vi "Demo.vi"() -> ()   [LabVIEW 2018]
uses:
  SquidstatStructures/AisDCData.ctl
  SquidstatStructures/AisACData.ctl
panel:
  in  "Start Experiment":bool
  in  "Experiment To Run":enum32{"DC Experiment", "AC Experiment"}(radio)
  out "Device Initialized?":bool
  in  "Channel To Run":i32
  in  "Stop Experiment":bool
  out "Experiment Active?":bool
  out "Last Channel":dbl
  out "Last AC Data":T1
  out "Last DC Data":T2
  out "Step Number":i32
  out "Step Name":string
  in  "Device Name":string
  # "Controls"
  # "Indicators"
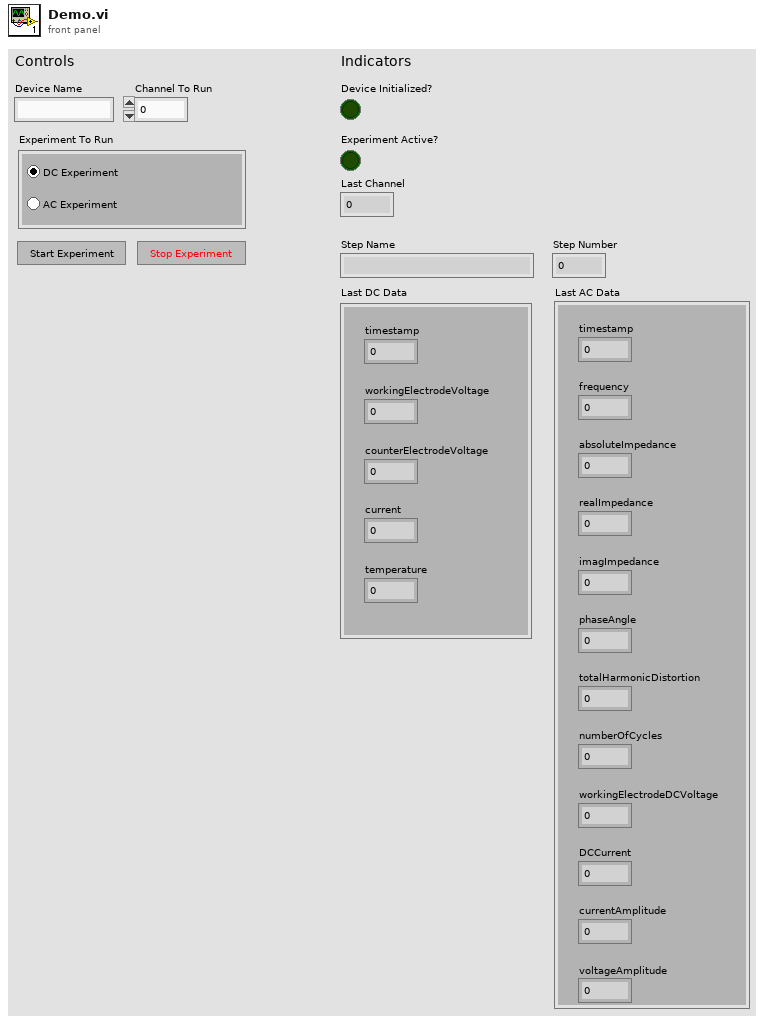
[diagram p1: front panel]
types:
  T1 = typedef "AisACData.ctl" = cluster{"timestamp":dbl, "frequency":dbl, "absoluteImpedance":dbl, "realImpedance":dbl, "imagImpedance":dbl, "phaseAngle":dbl, "totalHarmonicDistortion":dbl, "numberOfCycles":dbl, "workingElectrodeDCVoltage":dbl, "DCCurrent":dbl, "currentAmplitude":dbl, "voltageAmplitude":dbl}
  T2 = typedef "AisDCData.ctl" = cluster{"timestamp":dbl, "workingElectrodeVoltage":dbl, "counterElectrodeVoltage":dbl, "current":dbl, "temperature":dbl}
  T3 = typedef "AisUserEvents.ctl" = cluster{"Disconnected":refnum<user-event>, "Ground State":refnum<user-event>, "Device Error":refnum<user-event>, "New Element Started":refnum<user-event>, "Experiment Stopped":refnum<user-event>, "Experiment Paused":refnum<user-event>, "Experiment Resumed":refnum<user-event>, "DC Data":refnum<user-event>, "AC Data":refnum<user-event>}
  T4 = typedef "AisExperimentNode.ctl" = cluster{"Step Name":cluster{"char":u8, "char 2":u8, "char 3":u8, "char 4":u8, "char 5":u8, "char 6":u8, "char 7":u8, "char 8":u8, "char":u8, "char 9":u8, "char 10":u8, "char 11":u8, "char 12":u8, "char 13":u8, "char 14":u8, "char 15":u8, "char 16":u8, "char 17":u8, "char 18":u8, "char 19":u8, "char 20":u8, "char 21":u8, "char 22":u8, "char 23":u8, "char 24":u8, "char 25":u8, "char 26":u8, "char 27":u8, "char 28":u8, "char 29":u8, "char 30":u8, "char 31":u8, "char 32":u8, "char 33":u8, "char 34":u8, "char 35":u8, "char 36":u8, "char 37":u8, "char 38":u8, "char 39":u8, "char 40":u8, "char 41":u8, "char 42":u8, "char 43":u8, "char 44":u8, "char 45":u8, "char 46":u8, "char 47":u8, "char 48":u8, "char 49":u8, "char 50":u8, "char 50":u8}, "Step Number":i32, "Substep Number":i32, "Cycle Number":i32}
  T5 = cluster{"char":u8, "char 2":u8, "char 3":u8, "char 4":u8, "char 5":u8, "char 6":u8, "char 7":u8, "char 8":u8, "char":u8, "char 9":u8, "char 10":u8, "char 11":u8, "char 12":u8, "char 13":u8, "char 14":u8, "char 15":u8, "char 16":u8, "char 17":u8, "char 18":u8, "char 19":u8, "char 20":u8, "char 21":u8, "char 22":u8, "char 23":u8, "char 24":u8, "char 25":u8, "char 26":u8, "char 27":u8, "char 28":u8, "char 29":u8, "char 30":u8, "char 31":u8, "char 32":u8, "char 33":u8, "char 34":u8, "char 35":u8, "char 36":u8, "char 37":u8, "char 38":u8, "char 39":u8, "char 40":u8, "char 41":u8, "char 42":u8, "char 43":u8, "char 44":u8, "char 45":u8, "char 46":u8, "char 47":u8, "char 48":u8, "char 49":u8, "char 50":u8, "char 50":u8}
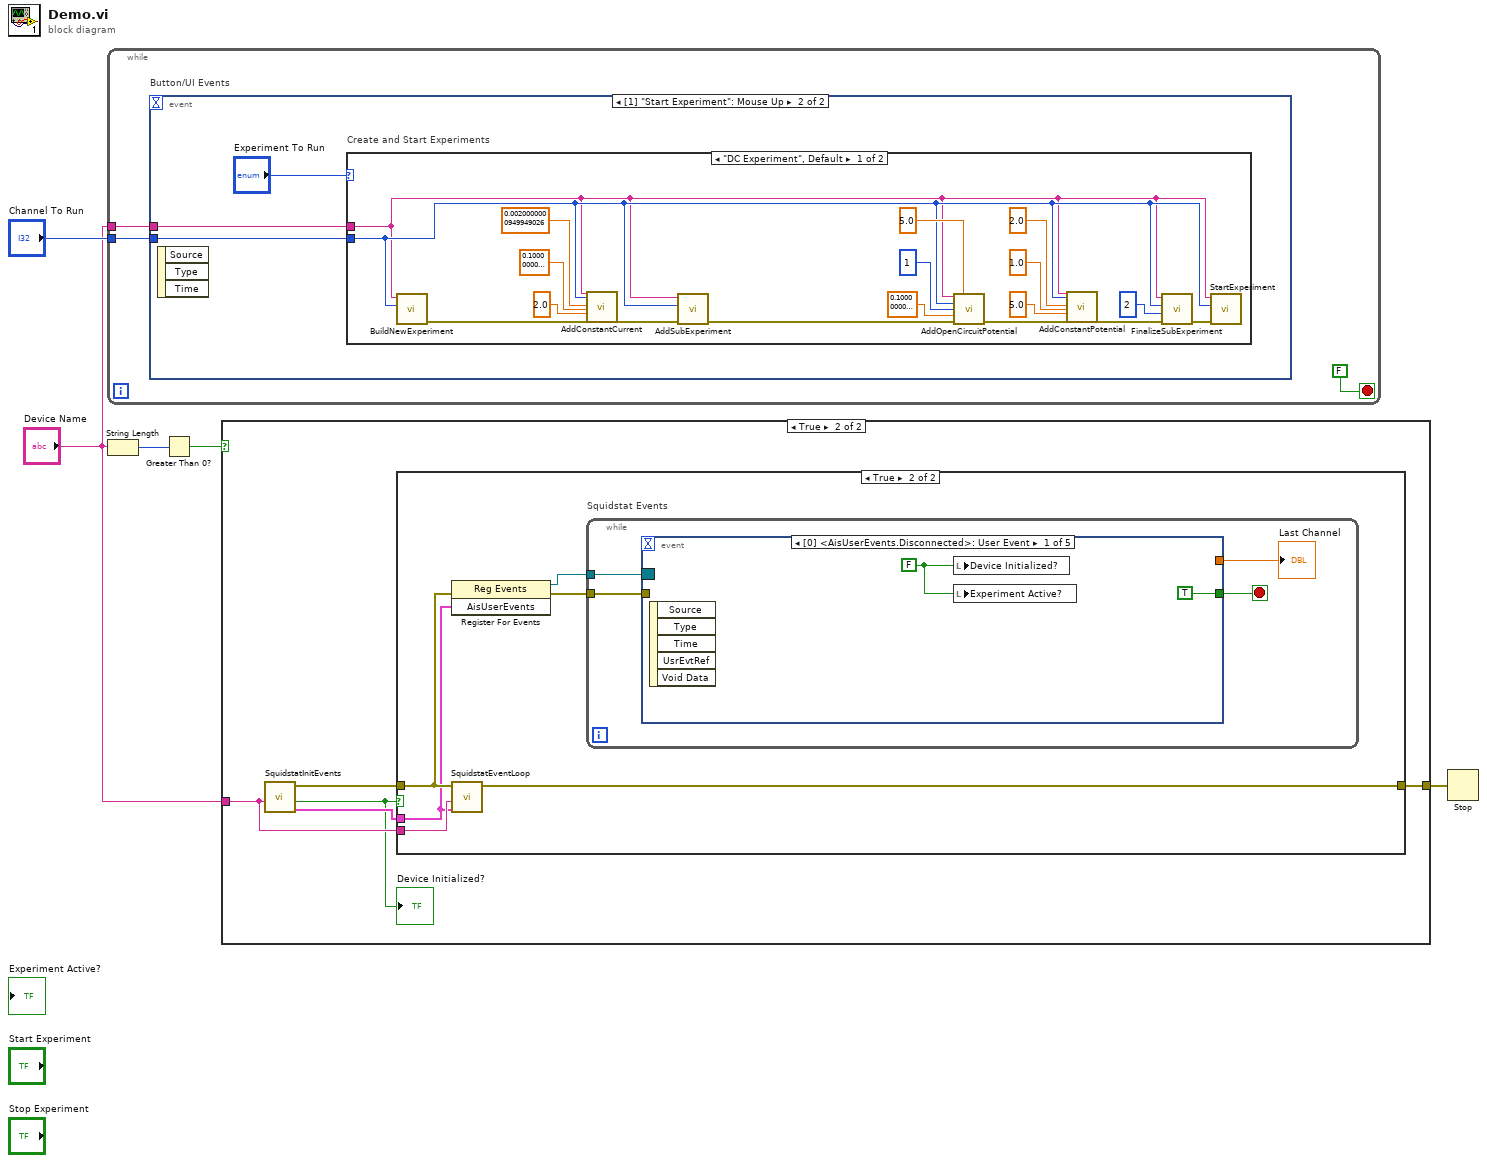
[diagram p0: block diagram]
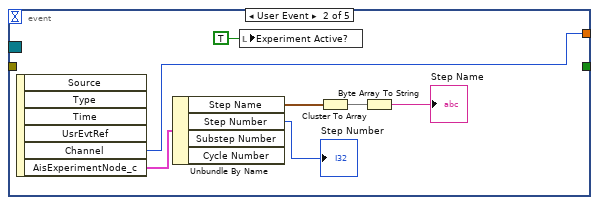
[diagram p4: hidden frame]
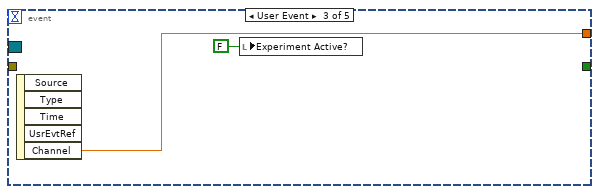
[diagram p5: hidden frame]
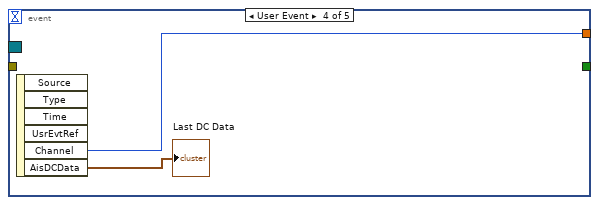
[diagram p6: hidden frame]
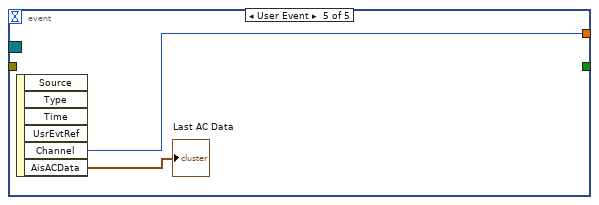
[diagram p7: hidden frame]
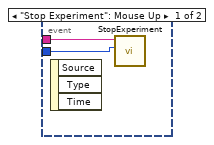
[diagram p8: hidden frame]
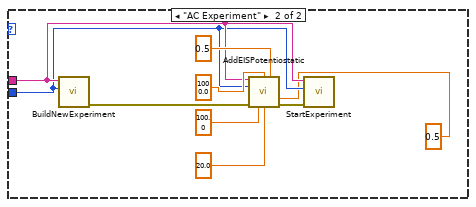
[diagram p9: hidden frame]
diagram:
  n1 = while {
    tunnel: "Device Name" -> [w8]
    tunnel: "Channel To Run" -> [w7]
    stop <- FALSE stop-if-true
    n2 = event "Button/UI Events" shown="[1] \"Start Experiment\": Mouse Up" {
      selector: _ -> [_ _]
      dyn-events: _ -> [_ _]
      timeout: _ -> [_ _]
      tunnel: w8 -> [w10 w11]
      tunnel: w7 -> [w9 w12]
      event "Stop Experiment": Mouse Up {
        n3 = event-data() -> ()  [unwired: 1 in, 3 out]
        n4 = call "StopExperiment.vi"("channel"=w9, "deviceName"=w10) -> ()  [unwired: 8 in, 2 out]
      }
      event "Start Experiment": Mouse Up {
        n5 = event-data() -> ()  [unwired: 1 in, 3 out]
        n6 = case "Create and Start Experiments" shown="\"DC Experiment\", Default" "Experiment To Run" {
          tunnel: w12 -> [w15 w33]
          tunnel: w11 -> [w14 w34]
          frame "DC Experiment", Default {
            n7 = call "BuildNewExperiment.vi"("channel"=w15, "deviceName"=w14) -> ("error out"=w31:errorcluster)  [unwired: 9 in]
            n8 = call "AddConstantCurrent.vi"("deviceName"=w14, "channel"=w15, "current"=sgl 0.002, "samplingInterval"=sgl 0.1, "maxDuration"=sgl 2.0, "error in (no error)"=w31) -> ("error out"=w24:errorcluster)  [unwired: 21 in]
            n9 = call "AddSubExperiment.vi"("error in (no error)"=w24, "channel"=w15, "deviceName"=w14) -> ("error out"=w23:errorcluster)  [unwired: 8 in]
            n10 = call "AddOpenCircuitPotential.vi"("deviceName"=w14, "maxDuration"=sgl 5.0, "channel"=w15, "repeats"=1, "samplingInterval"=sgl 0.1, "error in (no error)"=w23) -> ("error out"=w20:errorcluster)  [unwired: 9 in]
            n11 = call "AddConstantPotential.vi"("deviceName"=w14, "channel"=w15, "potential"=sgl 2.0, "samplingInterval"=sgl 1.0, "maxDuration"=sgl 5.0, "error in (no error)"=w20) -> ("error out"=w19:errorcluster)  [unwired: 21 in]
            n12 = call "FinalizeSubExperiment.vi"("error in (no error)"=w19, "repeats"=2, "channel"=w15, "deviceName"=w14) -> ("error out"=w22:errorcluster)  [unwired: 7 in]
            n13 = call "StartExperiment.vi"("error in (no error)"=w22, "channel"=w15, "deviceName"=w14) -> ()  [unwired: 7 in, 2 out]
          }
          frame "AC Experiment" {
            n14 = call "BuildNewExperiment.vi"("channel"=w33, "deviceName"=w34) -> ("error out"=w40:errorcluster)  [unwired: 9 in]
            n15 = call "AddEISPotentiostatic.vi"("deviceName"=w34, "endFreq"=sgl 1000.0, "biasVoltage"=sgl 0.5, "channel"=w33, "amplitude"=sgl 0.5, "error in (no error)"=w40, "startFreq"=sgl 100.0, "stepsPerDecade"=sgl 20.0) -> ("error out"=w39:errorcluster)  [unwired: 7 in]
            n16 = call "StartExperiment.vi"("error in (no error)"=w39, "channel"=w33, "deviceName"=w34) -> ()  [unwired: 7 in, 2 out]
          }
        }
      }
    }
  }
  n17 = String Length(string="Device Name") -> (length=w4:i32)
  n18 = Greater Than 0?(x=w4) -> (x > 0?=w1:bool)
  n19 = case shown="True" w1 {
    tunnel: "Device Name" -> [_ w43]
    tunnel: [_ w42] -> w2
    frame False {
    }
    frame True {
      n20 = call "SquidstatInitEvents.vi"("Device Name"=w43) -> ("AisUserEvents"=w44:T3, "Device OK"=w41:bool, "error out"=w45:errorcluster)  [unwired: 4 in]
      "Device Initialized?" <- w41
      n21 = case shown="True" w41 {
        tunnel: w44 -> [_ w49]
        tunnel: w45 -> [w46 w50]
        tunnel: w43 -> [_ w52]
        tunnel: [w46 w51] -> w42
        frame False {
        }
        frame True {
          n22 = register-events(error in=w50, w49) -> (reference out=w48:refnum<event-registration>, error out=w47:errorcluster)  [unwired: 1 in]
          n23 = call "SquidstatEventLoop.vi"("AisUserEvents"=w49, "Device Name"=w52, "error in (no error)"=w50) -> ("error out"=w51:errorcluster)  [unwired: 4 in]
          n24 = while "Squidstat Events" {
            tunnel: w48 -> [w54]
            tunnel: w47 -> [w55]
            stop <- w56 stop-if-true
            n25 = event shown="[0] <AisUserEvents.Disconnected>: User Event" {
              selector: w54 -> [_ _ _ _ _]
              dyn-events: _ -> [_ _ _ _ _]
              timeout: _ -> [_ _ _ _ _]
              tunnel: [TRUE _ _ _ _] -> w56
              tunnel: w55 -> [_ _ _ _ _]
              tunnel: [_ w60 w67 w68 w70] -> w53
              event User Event {
                w57 = FALSE
                n26 = event-data() -> ()  [unwired: 1 in, 5 out]
                n27 = local write "Device Initialized?"(w57) -> ()
                n28 = local write "Experiment Active?"(w57) -> ()
              }
              event User Event {
                n29 = event-data() -> ("Channel"=w60:u8, "AisExperimentNode_c"=w65:T4)  [unwired: 1 in, 4 out]
                n30 = Unbundle By Name(w65) -> ("Step Name"=w62:T5, "Step Number"=→"Step Number":i32)  [unwired: 2 out]
                n31 = local write "Experiment Active?"(TRUE) -> ()
                n32 = Cluster To Array(cluster=w62) -> (array=w61:u8[])
                n33 = Byte Array To String(unsigned byte array=w61) -> (string=→"Step Name":string)
              }
              event User Event {
                n34 = event-data() -> ("Channel"=w67:dbl)  [unwired: 1 in, 4 out]
                n35 = local write "Experiment Active?"(FALSE) -> ()
              }
              event User Event {
                n36 = event-data() -> ("Channel"=w68:u8, "AisDCData"=→"Last DC Data":T2)  [unwired: 1 in, 4 out]
              }
              event User Event {
                n37 = event-data() -> ("Channel"=w70:u8, "AisACData"=→"Last AC Data":T1)  [unwired: 1 in, 4 out]
              }
            }
            "Last Channel" <- w53
          }
        }
      }
    }
  }
  n38 = Stop(stop? (T)=w2) -> ()
